vi "INTERNSHIP PROJECT.vi"() -> ()   [LabVIEW 2018]
panel:
  out "your order will be prepared in":dbl
  in  "Pay bill and confirm":bool
  out "Discount":string
  out "Price 1":dbl
  in  "Quantity 1":dbl=1.0 min=1.0 max=10.0 step=1.0
  in  "item #1":bool
  out "Total,Bill":dbl
  out "Price 5":dbl
  in  "Quantity 5":dbl=1.0 min=1.0 max=10.0 step=1.0
  in  "item #1 5":bool
  out "Price 4":dbl
  in  "Quantity 4":dbl=1.0 min=1.0 max=10.0 step=1.0
  in  "item #1 4":bool
  out "Price 3":dbl
  in  "Quantity 3":dbl=1.0 min=1.0 max=10.0 step=1.0
  in  "item #1 3":bool
  in  "item #1 2":bool
  in  "Quantity 2":dbl=1.0 min=1.0 max=10.0 step=1.0
  out "Price 2":dbl
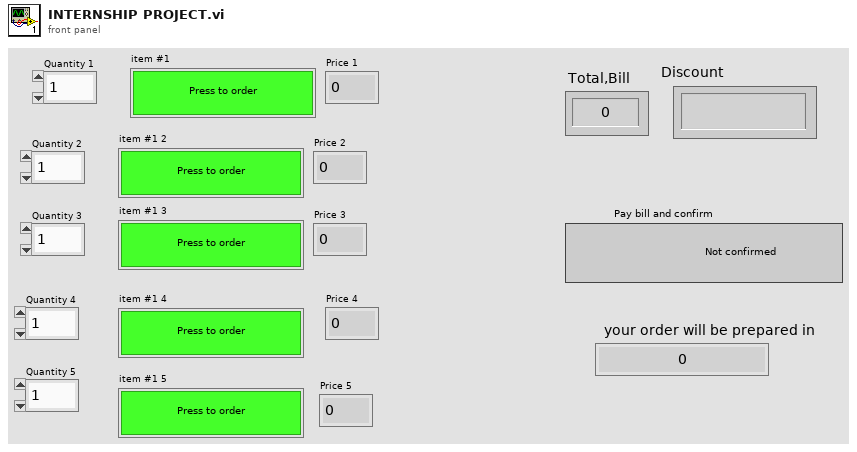
[diagram p1: front panel]
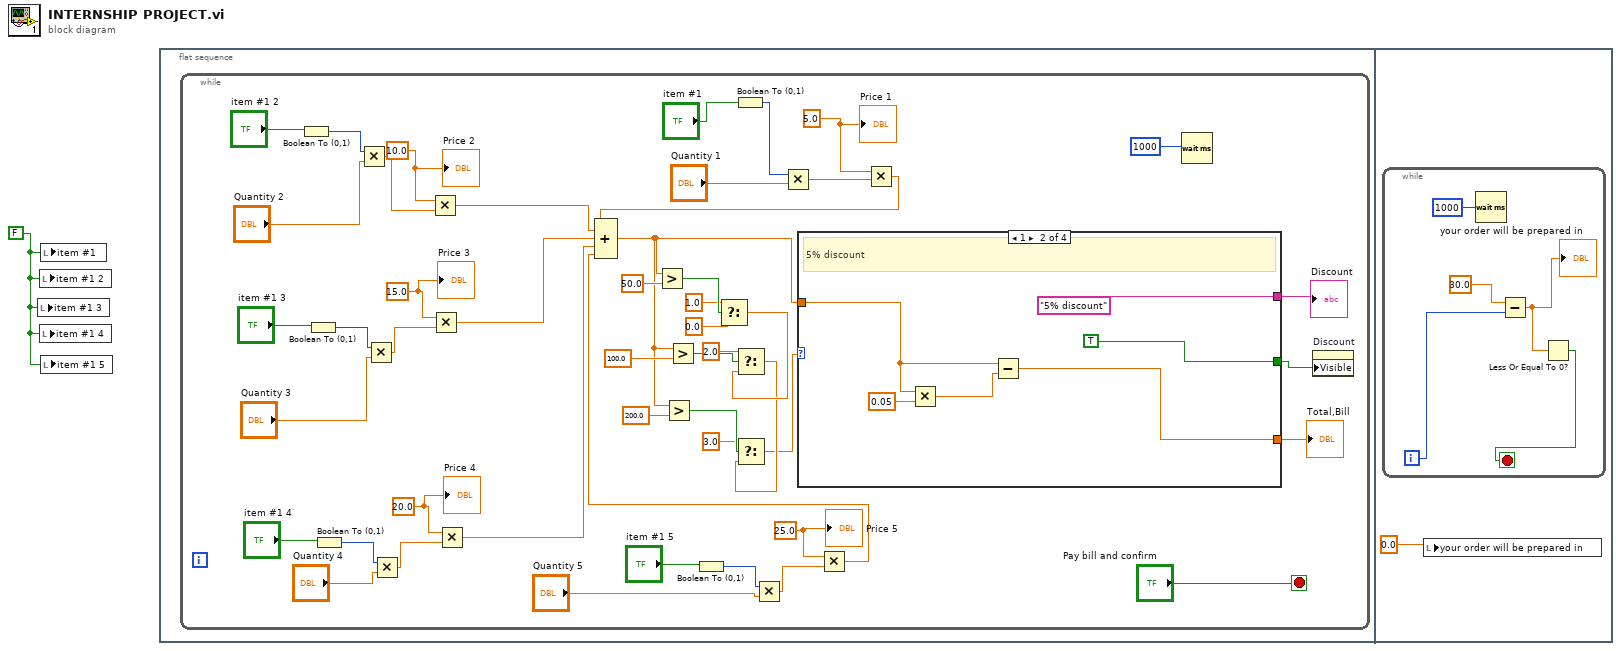
[diagram p0: block diagram]
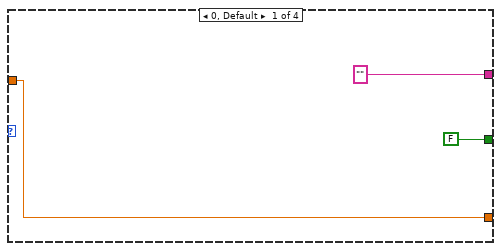
[diagram p2: hidden frame]
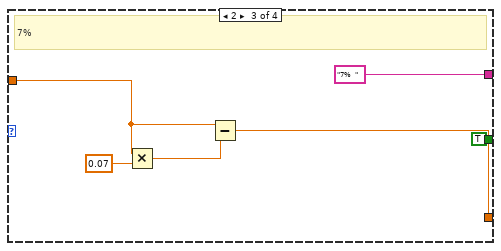
[diagram p3: hidden frame]
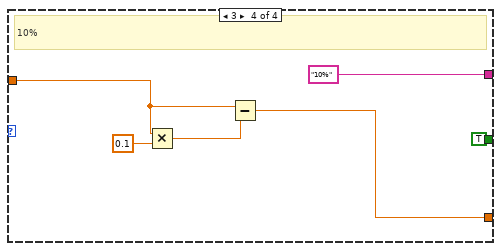
[diagram p4: hidden frame]
diagram:
  w1 = FALSE ("item #1")
  n1 = local write "item #1 3"(w1) -> ()
  n2 = local write "item #1 2"(w1) -> ()
  n3 = local write "item #1 4"(w1) -> ()
  n4 = local write "item #1"(w1) -> ()
  n5 = local write "item #1 5"(w1) -> ()
  n6 = flat-sequence {
    frame #0 {
      n7 = while {
        stop <- "Pay bill and confirm" stop-if-true
        w26 = 5.0 ("x")
        w28 = 25.0 ("x")
        w36 = 20.0 ("x")
        w41 = 15.0 ("x")
        w50 = 10.0 ("x")
        n8 = Boolean To (0,1)(Boolean="item #1 2") -> (0, 1=w47:i16)
        n9 = Boolean To (0,1)(Boolean="item #1 3") -> (0, 1=w44:i16)
        n10 = Boolean To (0,1)(Boolean="item #1 4") -> (0, 1=w39:i16)
        n11 = Multiply(x=w47, y="Quantity 2") -> (x*y=w49:dbl)
        n12 = Multiply(x=w44, y="Quantity 3") -> (x*y=w42:dbl)
        n13 = Multiply(x=w39, y="Quantity 4") -> (x*y=w37:dbl)
        n14 = Multiply(x=w50, y=w49) -> (x*y=w35:dbl)
        n15 = Multiply(x=w41, y=w42) -> (x*y=w34:dbl)
        n16 = Multiply(x=w36, y=w37) -> (x*y=w33:dbl)
        n17 = Boolean To (0,1)(Boolean="item #1 5") -> (0, 1=w31:i16)
        n18 = Boolean To (0,1)(Boolean="item #1") -> (0, 1=w23:i16)
        n19 = Multiply(x=w31, y="Quantity 5") -> (x*y=w29:dbl)
        n20 = Multiply(x=w23, y="Quantity 1") -> (x*y=w25:dbl)
        n21 = Multiply(x=w28, y=w29) -> (x*y=w27:dbl)
        n22 = Multiply(x=w26, y=w25) -> (x*y=w21:dbl)
        n23 = Compound Arithmetic op=ADD(w21, w35, w34, w33, w27) -> (w7:dbl)
        n24 = Greater?(x=w7, y=50.0) -> (0:w17:bool)
        n25 = Greater?(x=w7, y=200.0) -> (0:w11:bool)
        n26 = Greater?(x=w7, y=100.0) -> (0:w14:bool)
        n27 = Select(t=1.0, s=w17, f=0.0) -> (s? t:f=w12:dbl)
        n28 = Select(t=2.0, s=w14, f=w12) -> (s? t:f=w9:dbl)
        n29 = Select(t=3.0, s=w11, f=w9) -> (s? t:f=w8:dbl)
        n30 = case shown="1" w8 {
          tunnel: w7 -> [w53 w58 w63 w69]
          tunnel: [w53 w56 w62 w68] -> w6
          tunnel: ["" ("Discount") "5% discount" ("Discount") "7%  " ("Discount") "10%" ("Discount")] -> w5
          tunnel: [FALSE ("Visible") TRUE ("Visible") TRUE ("Visible") TRUE ("Visible")] -> w2
          frame 0, Default {
          }
          frame 1 {
            # "5% discount"
            n31 = Multiply(x=w58, y=0.05) -> (x*y=w57:dbl)
            n32 = Subtract(x=w58, y=w57) -> (x-y=w56:dbl)
          }
          frame 2 {
            # "7%"
            n33 = Multiply(x=w63, y=0.07) -> (x*y=w64:dbl)
            n34 = Subtract(x=w63, y=w64) -> (x-y=w62:dbl)
          }
          frame 3 {
            # "10%"
            n35 = Multiply(x=w69, y=0.1) -> (x*y=w70:dbl)
            n36 = Subtract(x=w69, y=w70) -> (x-y=w68:dbl)
          }
        }
        "Total,Bill" <- w6
        "Discount" <- w5
        n37 = Wait (ms)(milliseconds to wait=u32 1000) -> ()  [unwired: 1 out]
        n38 = property on="Discount" class="Str"("Visible"=w2) -> ()  [unwired: 2 in, 2 out]
        "Price 2" <- w50
        "Price 3" <- w41
        "Price 4" <- w36
        "Price 5" <- w28
        "Price 1" <- w26
      }
    }
    frame #1 {
      n39 = while {
        i -> [w76]
        stop <- w75 stop-if-true
        n40 = Wait (ms)(milliseconds to wait=u32 1000) -> ()  [unwired: 1 out]
        n41 = Subtract(x=30.0, y=w76) -> (x-y=w74:dbl)
        "your order will be prepared in" <- w74
        n42 = Less Or Equal To 0?(x=w74) -> (x <= 0?=w75:bool)
      }
      n43 = local write "your order will be prepared in"(0.0 ("your order will be prepared in")) -> ()
    }
  }
